vi "File to Array.vi"(8 "error in":errorcluster, 11 "file path in":path) -> (0 "error out":errorcluster, 2 "list out":T1[](array[typedef]) {"Creation Date" format="%<%x>T"; "Last Updated" format="%<%x>T"}, 3 "file path out":path)   [LabVIEW 2018]
uses:
  Type Defs/SR Cluster.ctl
  Type Defs/SR Status.ctl
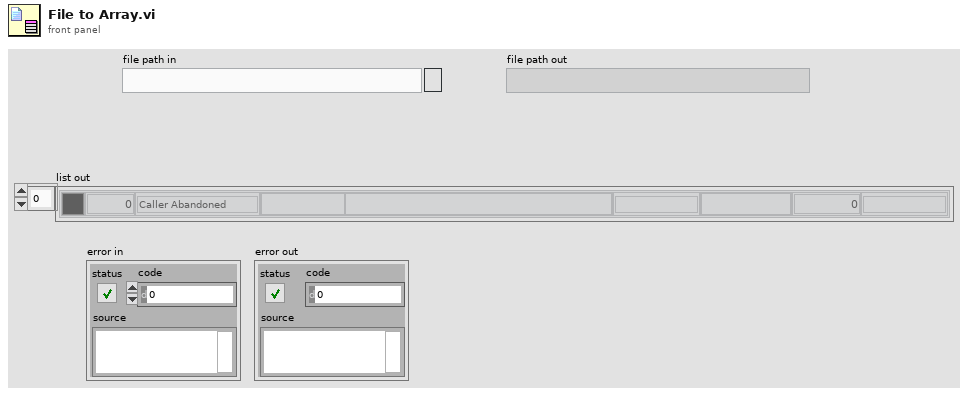
[diagram p1: front panel]
types:
  T1 = typedef "SR Cluster.ctl" = cluster{"Color":u32, "SR Number":i32, "SR Status":T2, "SR Type":string, "Summary":string, "Last Updated":timestamp, "Service Level":string, "Days Open":dbl, "Creation Date":timestamp}
  T2 = typedef "SR Status.ctl" = enum16{"Caller Abandoned", "Created in Error", "Expired", "Forum Resolved AE", "Forum Resolved Customer", "IN WORK", "IN WORK Collab with AES", "IN WORK Collab with PSE", "IN WORK Collab with SE", "IN WORK Customer Added Note", "IN WORK Escalation", "IN WORK Wait on Customer", "Open", "Potentially Resolved", "Presumed Resolved", "RMA Approved for Return", "Resolved", "Passed Off"}
  T3 = enum16{"open", "replace", "create", "open or create", "replace or create", "replace or create with confirmation"}
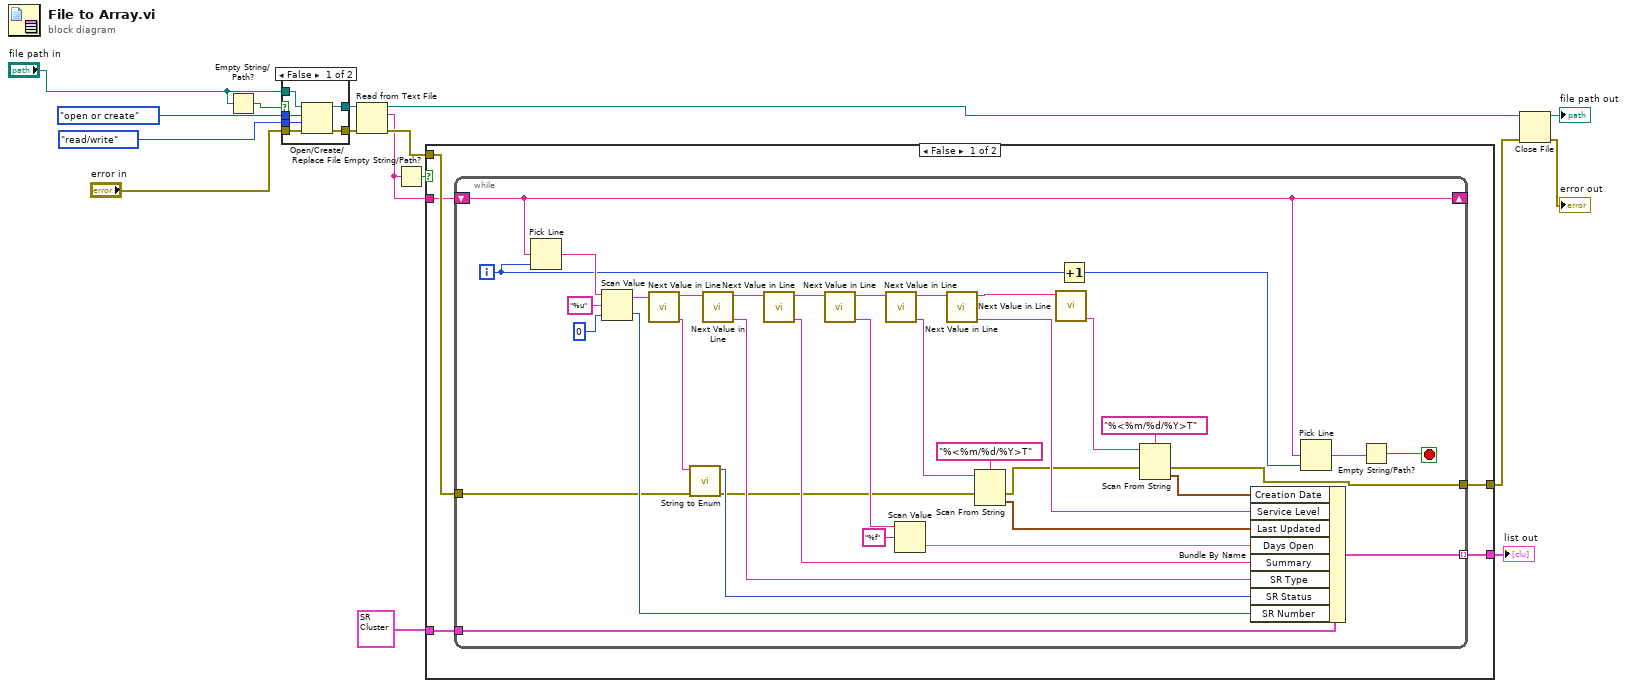
[diagram p0: block diagram]
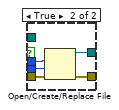
[diagram p2: hidden frame]
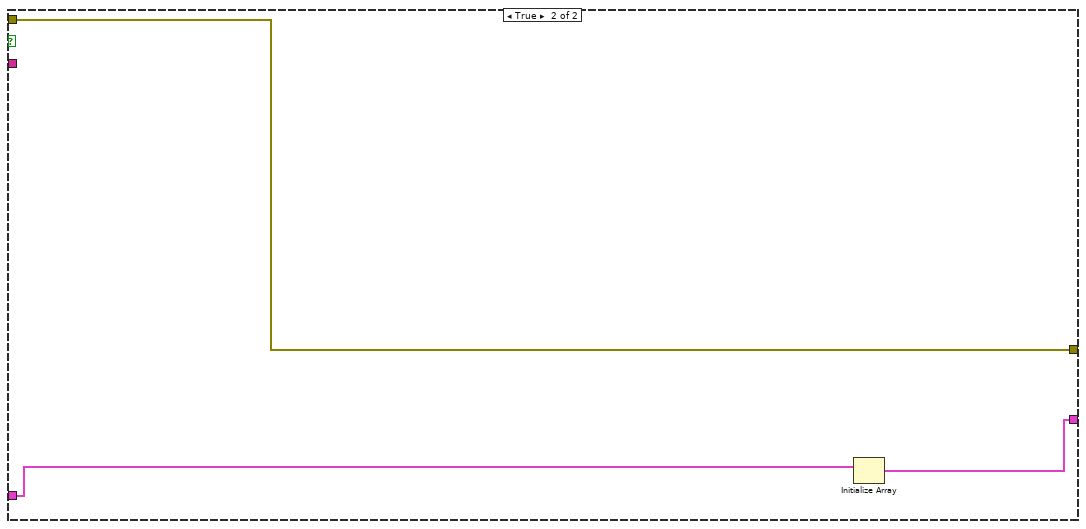
[diagram p3: hidden frame]
diagram:
  n1 = Empty String/Path?(string/path="file path in") -> (empty?=w2:bool)
  n2 = case shown="False" w2 {
    tunnel: enum16{"read/write", "read-only", "write-only"}."read/write" ("access (0:read/write)") -> [w22 w26]
    tunnel: T3."open or create" ("operation (0:open)") -> [w21 w27]
    tunnel: "error in" -> [w20 w25]
    tunnel: [w19 w23] -> w13
    tunnel: [w18 w24] -> w12
    tunnel: "file path in" -> [w17 _]
    frame False {
      n3 = Open/Create/Replace File(file path (use dialog)=w17, error in=w20, operation (0:open)=w21, access (0:read/write)=w22) -> (refnum out=w19:refnum<file>, error out=w18:errorcluster)  [unwired: 2 in, 1 out]
    }
    frame True {
      n4 = Open/Create/Replace File(error in=w25, operation (0:open)=w27, access (0:read/write)=w26) -> (refnum out=w23:refnum<file>, error out=w24:errorcluster)  [unwired: 3 in, 1 out]
    }
  }
  n5 = Read from Text File(file (use dialog)=w13, error in=w12) -> (refnum out=w7:refnum<file>, text=w9:string, error out=w10:errorcluster)  [unwired: 2 in, 1 out]
  n6 = Empty String/Path?(string/path=w9) -> (empty?=w11:bool)
  n7 = case shown="False" w11 {
    tunnel: w10 -> [w31 w69]
    tunnel: w9 -> [w30 _]
    tunnel: T1 {"Color"=0, "SR Number"=0, "SR Status"=enum."Caller Abandoned", "SR Type"="", "Summary"="", "Last Updated"=timestamp(0 s since 1904-01-01), "Service Level"="", "Days Open"=0.0, "Creation Date"=timestamp(0 s since 1904-01-01)} ("SR Cluster") -> [w32 w71]
    tunnel: [w29 w69] -> w6
    tunnel: [w28 w70] -> w5
    frame False {
      n8 = while {
        tunnel: w32 -> [w59]
        tunnel: w31 -> [w40]
        shift-right: [w47] -> _
        shift-left: w30 -> [w47]
        tunnel: [w48] -> w28 mode=indexing
        tunnel: [w33] -> w29
        i -> [w44]
        stop <- w45 stop-if-true
        n9 = Pick Line(multi-line string=w47, line index=w44) -> (output string=w68:string)  [unwired: 1 in]
        n10 = Scan Value(string=w68, format string="%u", default (0 dbl)=0) -> (output string=w65:string, value=w58:i32)
        n11 = call "Next Value in Line.vi"("string in"=w65) -> ("value"=w42:string, "rest of string"=w64:string)  [unwired: 9 in]
        n12 = call "String to Enum.vi"("error in"=w40, "string in"=w42) -> ("error out"=w39:errorcluster, "enum out"=w41:T2)  [unwired: 8 in]
        n13 = call "Next Value in Line.vi"("string in"=w64) -> ("value"=w57:string, "rest of string"=w63:string)  [unwired: 9 in]
        n14 = call "Next Value in Line.vi"("string in"=w63) -> ("value"=w56:string, "rest of string"=w62:string)  [unwired: 9 in]
        n15 = call "Next Value in Line.vi"("string in"=w62) -> ("value"=w54:string, "rest of string"=w61:string)  [unwired: 9 in]
        n16 = call "Next Value in Line.vi"("string in"=w61) -> ("value"=w52:string, "rest of string"=w60:string)  [unwired: 9 in]
        n17 = Scan Value(string=w54, format string="%f") -> (value=w55:dbl)  [unwired: 1 in, 1 out]
        n18 = call "Next Value in Line.vi"("string in"=w60) -> ("value"=w49:string, "rest of string"=w38:string)  [unwired: 9 in]
        n19 = Scan From String(format string="%<%m/%d/%Y>T", input string=w52, error in=w39) -> (error out=w34:errorcluster, output 1=w50:timestamp)  [unwired: 2 in, 2 out]
        n20 = call "Next Value in Line.vi"("string in"=w38) -> ("value"=w37:string)  [unwired: 9 in, 1 out]
        n21 = Increment(x=w44) -> (x+1=w43:i32)
        n22 = Scan From String(format string="%<%m/%d/%Y>T", input string=w37, error in=w34) -> (error out=w33:errorcluster, output 1=w35:timestamp)  [unwired: 2 in, 2 out]
        n23 = Bundle By Name(cluster=w59, "Creation Date"=w35, "Service Level"=w49, "Last Updated"=w50, "Days Open"=w55, "Summary"=w56, "SR Type"=w57, "SR Status"=w41, "SR Number"=w58) -> (w48:T1)
        n24 = Pick Line(multi-line string=w47, line index=w43) -> (output string=w46:string)  [unwired: 1 in]
        n25 = Empty String/Path?(string/path=w46) -> (empty?=w45:bool)
      }
    }
    frame True {
      n26 = Initialize Array(w71) -> (w70:T1[])  [unwired: 1 in]
    }
  }
  "list out" <- w5
  n27 = Close File(refnum=w7, error in=w6) -> (path=→"file path out":path, error out=→"error out":errorcluster)
